vi "Initialize Hardware References.vi"(8 "error in (no error)":errorcluster, 11 "Hardware Resources in":T1) -> (0 "error out":errorcluster, 3 "Hardware Resources out":T1)   [LabVIEW 2013, in "Logging Acquisition.lvlib"]
doc: "Initialize the hardware references."
uses:
  Logging Acquisition.lvlib
  Hardware Configuration.ctl
  Signal Type.ctl
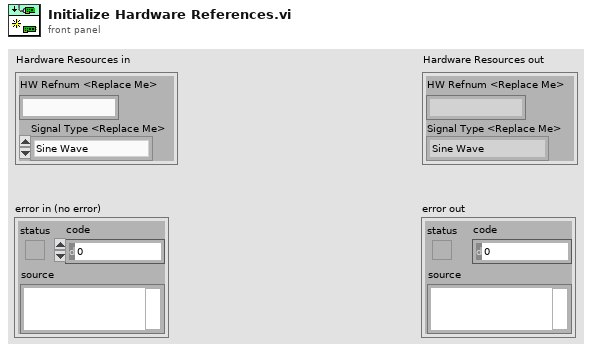
[diagram p1: front panel]
types:
  T1 = typedef "Logging Acquisition.lvlib/Hardware Configuration.ctl" = cluster{"HW Refnum <Replace Me>":string, "Signal Type <Replace Me>":T2}
  T2 = typedef "Logging Acquisition.lvlib/Signal Type.ctl" = enum16{"Sine Wave", "Square with Noise"}
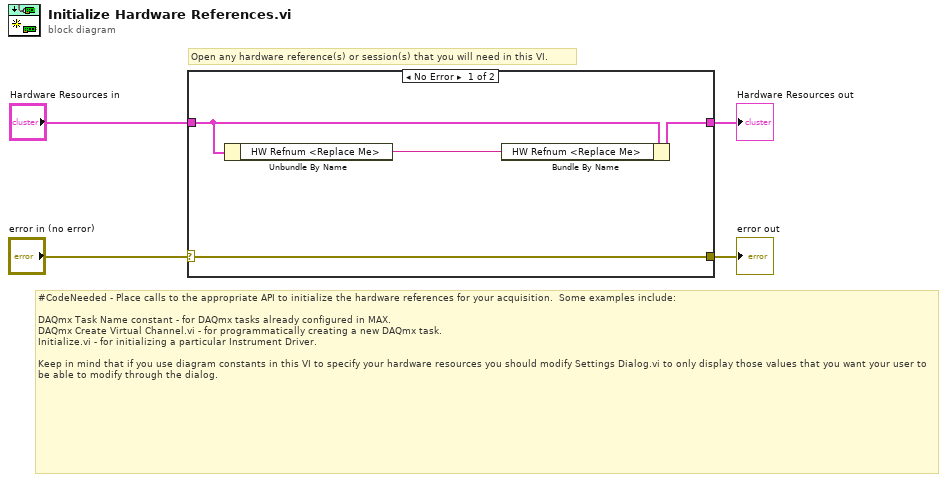
[diagram p0: block diagram]
diagram:
  # "Open any hardware reference(s) or session(s) that you will need in this VI."
  # "#CodeNeeded - Place calls to the appropriate API to initialize the hardware references for your acquisition.  Some examples include:\n\nDAQmx Task Name constant - for DAQmx tasks already configured in MAX.\nDAQmx Create Virtual Channel.vi - for programmatically creating a new DAQmx task.\nInitialize.vi - for initializing a particular Instrument Driver.\n\nKeep in mind that if you use diagram constants in this VI to specify your hardware resources you should modify Settings Dialog.vi to only display those values that you want your user to be able to modify through the dialog."
  n1 = case shown="No Error" "error in (no error)" {
    selector: "error in (no error)" -> [w7 w9]
    tunnel: [w7 w9] -> w3
    tunnel: "Hardware Resources in" -> [w6 w10]
    tunnel: [w8 w10] -> w1
    frame No Error {
      n2 = Unbundle By Name(w6) -> ("HW Refnum <Replace Me>"=w5:string)
      n3 = Bundle By Name(cluster=w6, "HW Refnum <Replace Me>"=w5) -> (w8:T1)
    }
    frame Error {
    }
  }
  "Hardware Resources out" <- w1
  "error out" <- w3
